vi "Main_08a refactored.vi"() -> ()   [LabVIEW 2020]
panel:
  out "Puzzle Array":i32[][](array[numeric])
  out "sum":u32
  in  "Puzzle":string="200200221023111313131033314121142013103432145142351212334232423210101340410243413011333312111010010\n021002023301222221234134021422342024344555521535143232341414552024224120114233210330203002020100112\n120000123021210023111321143114331115334535223455511513445233523154411102203411040133312002213001021\n110211312303200204232110124204135453554533435152342542252215415141133330323032234114310011301232202\n112002122201001100330432244432552555524445123151222142521452233321152332132412434434431321322021220\n000131233030332102140440124221314455255431113413445553414144524134315351524134030112312012102102122\n..."
  in  "Example":string="30373\n25512\n65332\n33549\n35390"
  # "--- Day 8: Treetop Tree House ---\nThe expedition comes across a peculiar patch of tall trees all planted carefully in a grid. The Elves explain that a previous expedition planted these trees as a reforestation effort. Now, they're curious if this would be a good location for a tree house.\n\nFirst, determine whether there is enough tree cover here to keep a tree house hidden. To do this, you need to count the number of trees that are visible from outside the grid when looking directly along a row or column.\n\nThe Elves have already launched a quadcopter to generate a map with the height of each tree (your puzzle input). For example:\n\n30373\n25512\n65332\n33549\n35390\nEach tree is represented as a single digit whose value is its height, where 0 is the shortest and 9 is the tallest.\n\nA tree is visible if all of the other trees between it and an edge of the grid are shorter than it. Only consider trees in the same row or column; that is, only look up, down, left, or right from any given tree.\n\nAll of the trees around the edge of the grid are visible - since they are already on the edge, there are no trees to block the view. In this example, that only leaves the interior nine trees to consider:\n\nThe top-left 5 is visible from the left and top. (It isn't visible from the right or bottom since other trees of height 5 are in the way.)\nThe top-middle 5 is visible from the top and right.\nThe top-right 1 is not visible from any direction; for it to be visible, there would need to only be trees of height 0 between it and an edge.\nThe left-middle 5 is visible, but only from the right.\nThe center 3 is not visible from any direction; for it to be visible, there would need to be only trees of at most height 2 between it and an edge.\nThe right-middle 3 is visible from the right.\nIn the bottom row, the middle 5 is visible, but the 3 and 4 are not.\nWith 16 trees visible on the edge and another 5 visible in the interior, a total of 21 trees are visible in this arrangement.\n\nConsider your map; how many trees are visible from outside the grid?"
  # "1818"
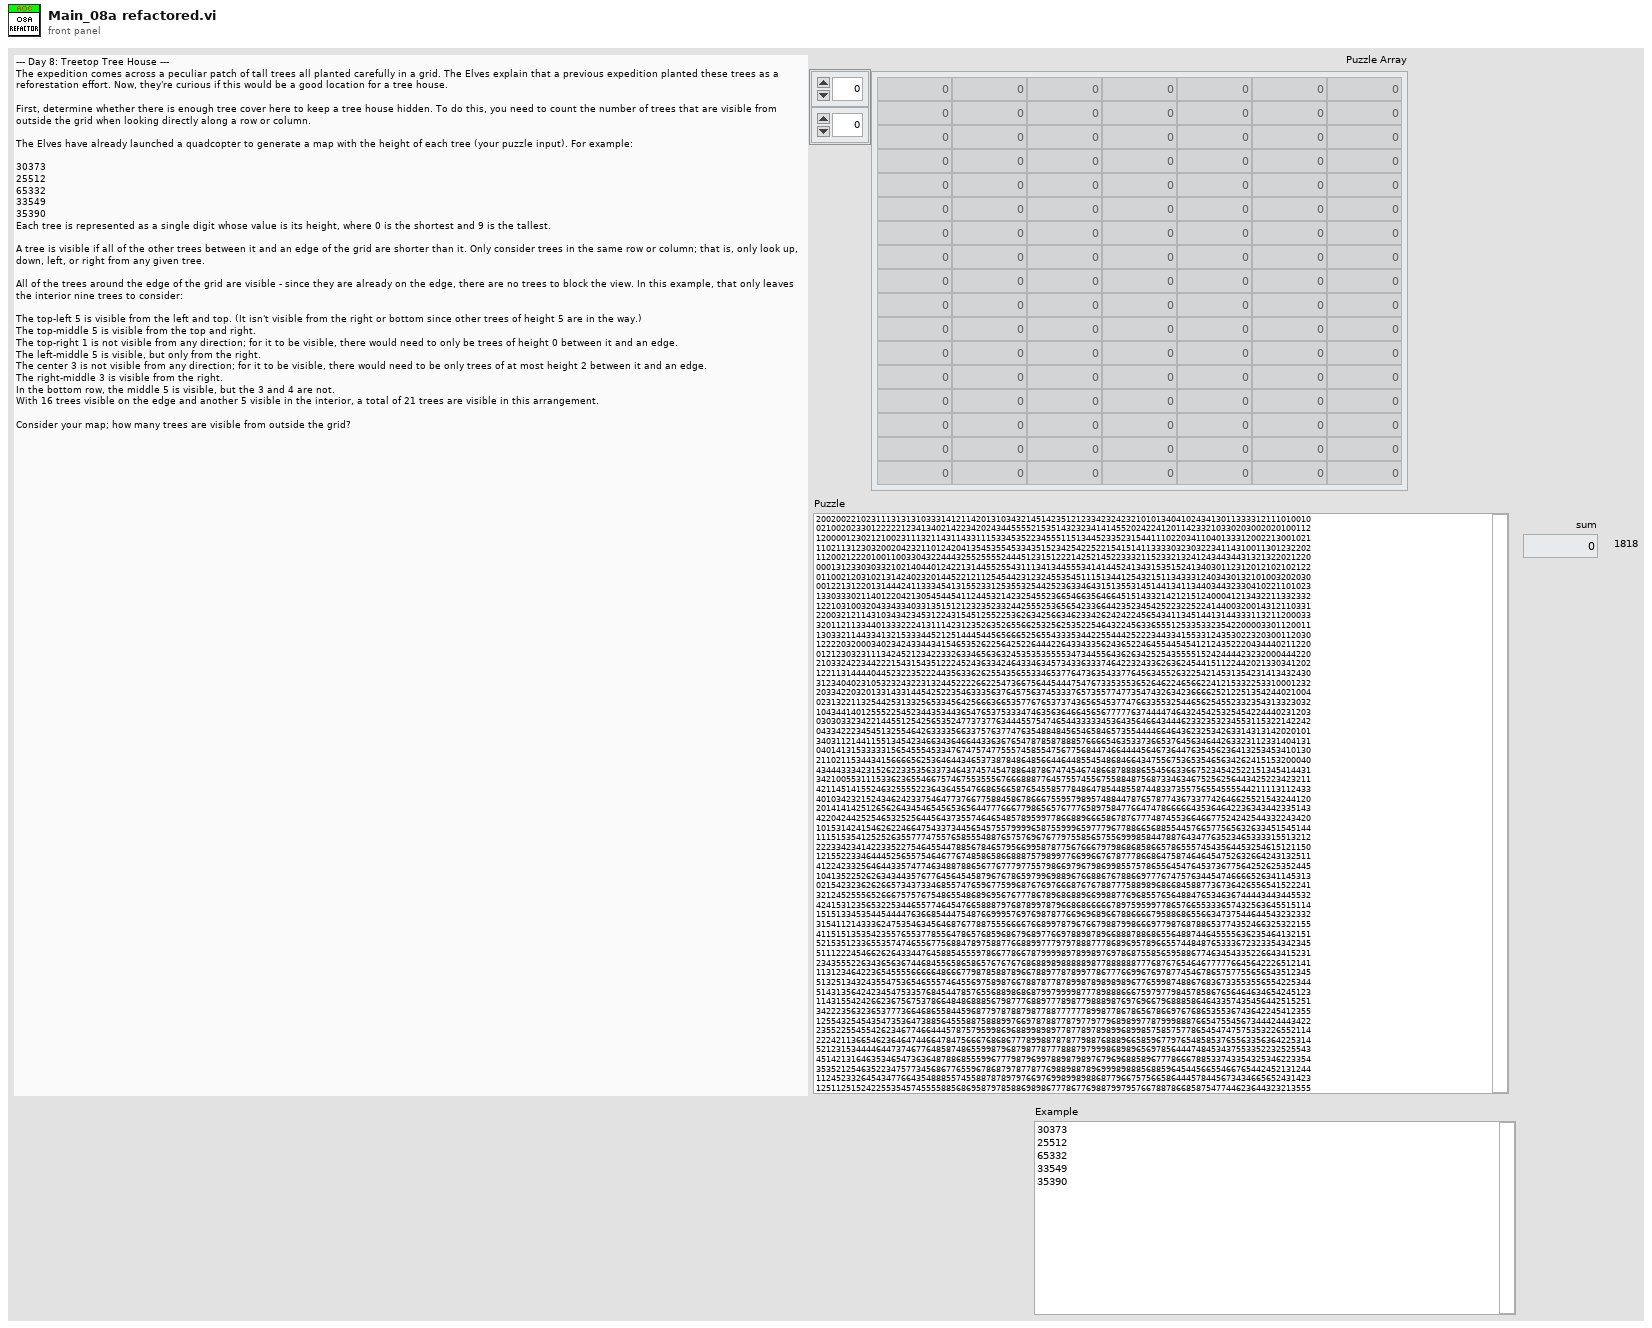
[diagram p1: front panel]
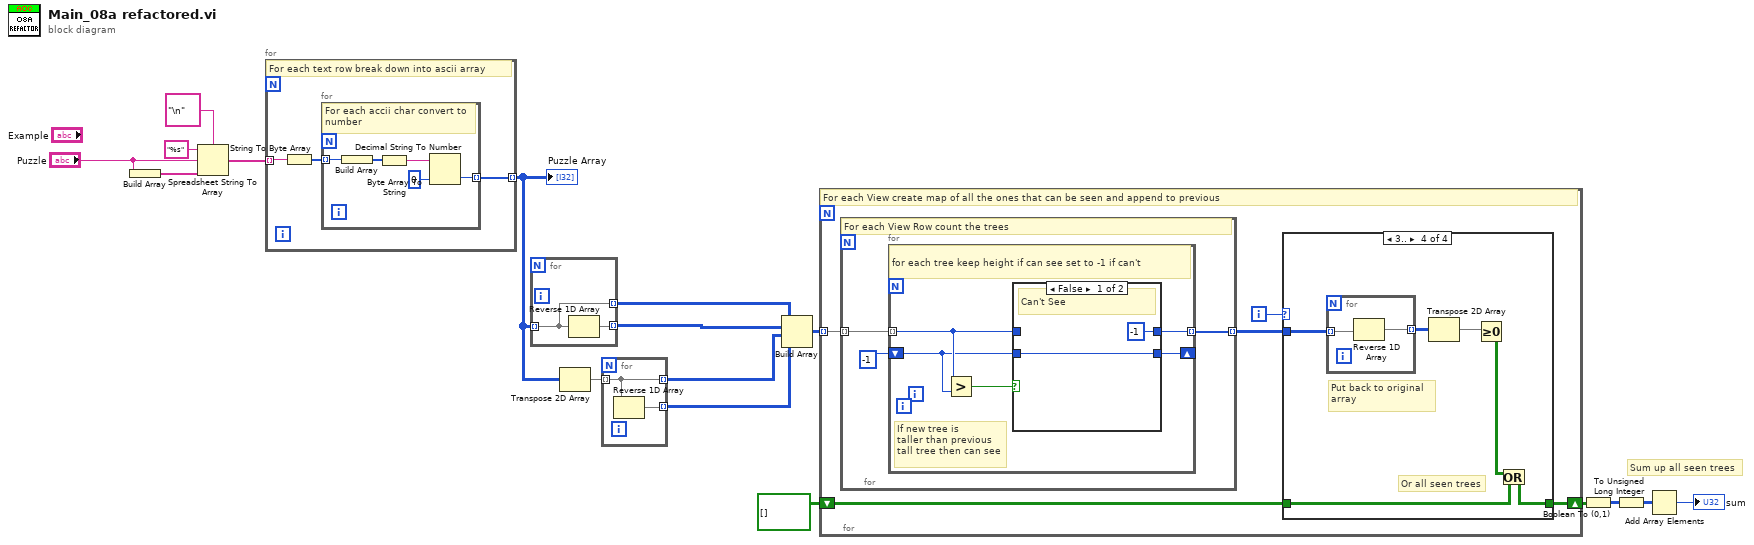
[diagram p0: block diagram]
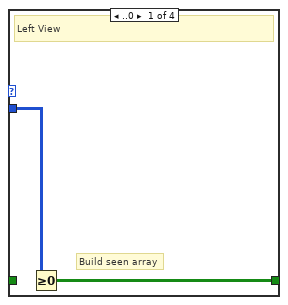
[diagram p2: hidden frame]
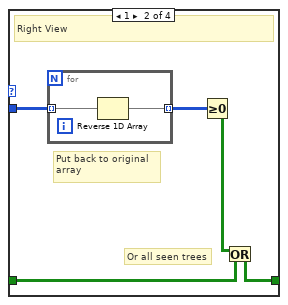
[diagram p3: hidden frame]
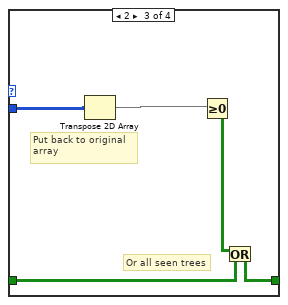
[diagram p4: hidden frame]
diagram:
  # "Sum up all seen trees"
  n1 = Build Array("Puzzle") -> (w12:string[])
  n2 = Spreadsheet String To Array(delimiter (Tab)="\n", format string="%s", spreadsheet string="Puzzle", array type (2D Dbl)=w12) -> (array=w9:string[])
  n3 = for {
    tunnel: w9 -> [w20] mode=indexing
    tunnel: [w18] -> w8 mode=indexing
    # "For each text row break down into ascii array"
    n4 = String To Byte Array(string=w20) -> (unsigned byte array=w19:u8[])
    n5 = for {
      tunnel: w19 -> [w25] mode=indexing
      tunnel: [w21] -> w18 mode=indexing
      # "For each accii char convert to number"
      n6 = Build Array(w25) -> (w24:u8[])
      n7 = Byte Array To String(unsigned byte array=w24) -> (string=w23:string)
      n8 = Decimal String To Number(string=w23, default (0L)=0 ("default (0 I32)")) -> (number=w21:i32)  [unwired: 1 in, 1 out]
    }
  }
  "Puzzle Array" <- w8
  n9 = for {
    tunnel: w8 -> [w26] mode=indexing
    tunnel: [w27] -> w5 mode=indexing
    tunnel: [w26] -> w6 mode=indexing
    n10 = Reverse 1D Array(array=w26) -> (reversed array=w27:i32[])
  }
  n11 = Transpose 2D Array(2D array=w8) -> (transposed array=w7:i32[][])
  n12 = for {
    tunnel: w7 -> [w28] mode=indexing
    tunnel: [w29] -> w3 mode=indexing
    tunnel: [w28] -> w4 mode=indexing
    n13 = Reverse 1D Array(array=w28) -> (reversed array=w29:i32[])
  }
  n14 = Build Array(w6, w5, w4, w3) -> (w1:i32[][][])
  n15 = for {
    tunnel: w1 -> [w34] mode=indexing
    shift-right: [w32] -> w17
    shift-left: bool[][] [] -> [w31]
    i -> [w33]
    # "For each View create map of all the ones that can be seen and append to previous"
    n16 = for {
      tunnel: w34 -> [w59] mode=indexing
      tunnel: [w57] -> w30 mode=indexing
      # "For each View Row count the trees"
      n17 = for {
        tunnel: w59 -> [w63] mode=indexing
        shift-right: [w61] -> _
        shift-left: -1 -> [w60]
        tunnel: [w62] -> w57 mode=indexing
        # "If new tree is \ntaller than previous\ntall tree then can see"
        # "for each tree keep height if can see set to -1 if can't"
        n18 = Greater?(x=w63, y=w60) -> (0:w64:bool)
        n19 = case shown="False" w64 {
          tunnel: w63 -> [_ w67]
          tunnel: [-1 w67] -> w62
          tunnel: [w65 w67] -> w61
          tunnel: w60 -> [w65 _]
          frame False {
            # "Can't See"
          }
          frame True {
            # "Can See"
          }
        }
      }
    }
    n20 = case shown="3.." w33 {
      tunnel: [w36 w40 w47 w53] -> w32
      tunnel: w31 -> [_ w41 w48 w54]
      tunnel: w30 -> [w35 w38 w45 w51]
      frame ..0 {
        # "Build seen array"
        # "Left View"
        n21 = Greater Or Equal To 0?(x=w35) -> (x >= 0?=w36:bool[][])
      }
      frame 1 {
        # "Or all seen trees"
        # "Put back to original\narray"
        # "Right View"
        n22 = for {
          tunnel: w38 -> [w43] mode=indexing
          tunnel: [w42] -> w37 mode=indexing
          n23 = Reverse 1D Array(array=w43) -> (reversed array=w42:i32[])
        }
        n24 = Greater Or Equal To 0?(x=w37) -> (x >= 0?=w39:bool[][])
        n25 = Or(x=w39, y=w41) -> (x .or. y?=w40:bool[][])
      }
      frame 2 {
        # "Or all seen trees"
        # "Put back to original\narray"
        n26 = Transpose 2D Array(2D array=w45) -> (transposed array=w44:i32[][])
        n27 = Greater Or Equal To 0?(x=w44) -> (x >= 0?=w46:bool[][])
        n28 = Or(x=w46, y=w48) -> (x .or. y?=w47:bool[][])
      }
      frame 3.. {
        # "Or all seen trees"
        # "Put back to original\narray"
        n29 = for {
          tunnel: w51 -> [w56] mode=indexing
          tunnel: [w55] -> w50 mode=indexing
          n30 = Reverse 1D Array(array=w56) -> (reversed array=w55:i32[])
        }
        n31 = Transpose 2D Array(2D array=w50) -> (transposed array=w49:i32[][])
        n32 = Greater Or Equal To 0?(x=w49) -> (x >= 0?=w52:bool[][])
        n33 = Or(x=w52, y=w54) -> (x .or. y?=w53:bool[][])
      }
    }
  }
  n34 = Boolean To (0,1)(Boolean=w17) -> (0, 1=w16:i16[][])
  n35 = To Unsigned Long Integer(number=w16) -> (unsigned 32bit integer=w14:u32[][])
  n36 = Add Array Elements(numeric array=w14) -> (sum=→"sum":u32)
